vi "TeleopEnqueueInput.vi"(8 "error in (no error)":errorcluster, 10 "Variant":variant, 11 "QueueEnum":T1) -> (0 "error out":errorcluster)   [LabVIEW 2012]
uses:
  QueueEnum.ctl
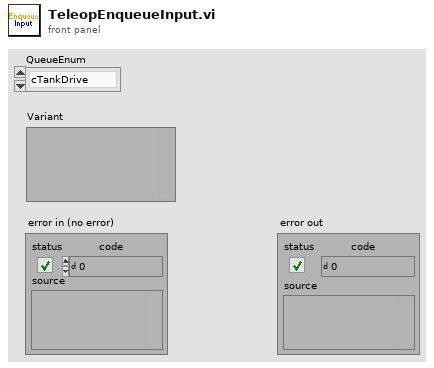
[diagram p1: front panel]
types:
  T1 = typedef "QueueEnum.ctl" = enum16{"cTankDrive", "cClimb", "cLauncherAngle", "cLauncherWheel", "cFirePneumatic"}
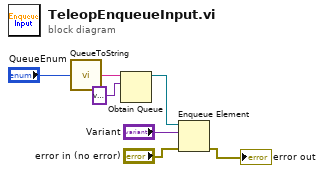
[diagram p0: block diagram]
diagram:
  n1 = call "QueueToString.vi"("QueueEnum"="QueueEnum") -> ("String"=w4:string)
  n2 = Obtain Queue(name (unnamed)=w4, element data type=variant) -> (queue out=w1:refnum<queue>)  [unwired: 3 in, 2 out]
  n3 = Enqueue Element(queue=w1, element="Variant", error in (no error)="error in (no error)") -> (error out=→"error out":errorcluster)  [unwired: 1 in, 2 out]
